vi "DualGateSTS.vi"() -> ()   [LabVIEW 2021]
panel:
  in  "Tabs":enum32{"Main", "Attributes"}(tab)
  in  "Start Gate 1 (V)":dbl
  in  "End Gate 1 (V)":dbl
  in  "Increment Gate 1 (V)":dbl
  in  "Safety Limit 2 (V)":dbl
  in  "Basename":string
  in  "Start Gate 2 (V)":dbl
  in  "End Gate 2 (V)":dbl
  in  "Increment Gate 2 (V)":dbl
  in  "Stop":bool
  out "Current Gate Voltage 2 (V)":dbl
  in  "Attributes":string[][](array[string])
  # "Dual Gate STS"
  # "Gate 2 Parameters"
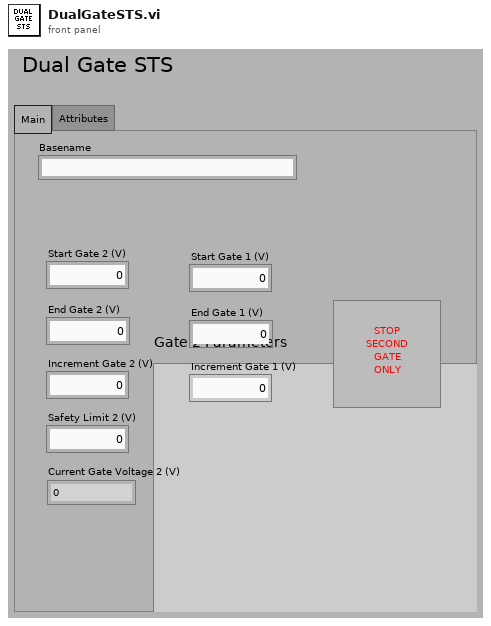
[diagram p1: front panel]
types:
  T1 = enum16{"Output 2 (V)", "Output 3 (V)", "Output 4 (V)"}
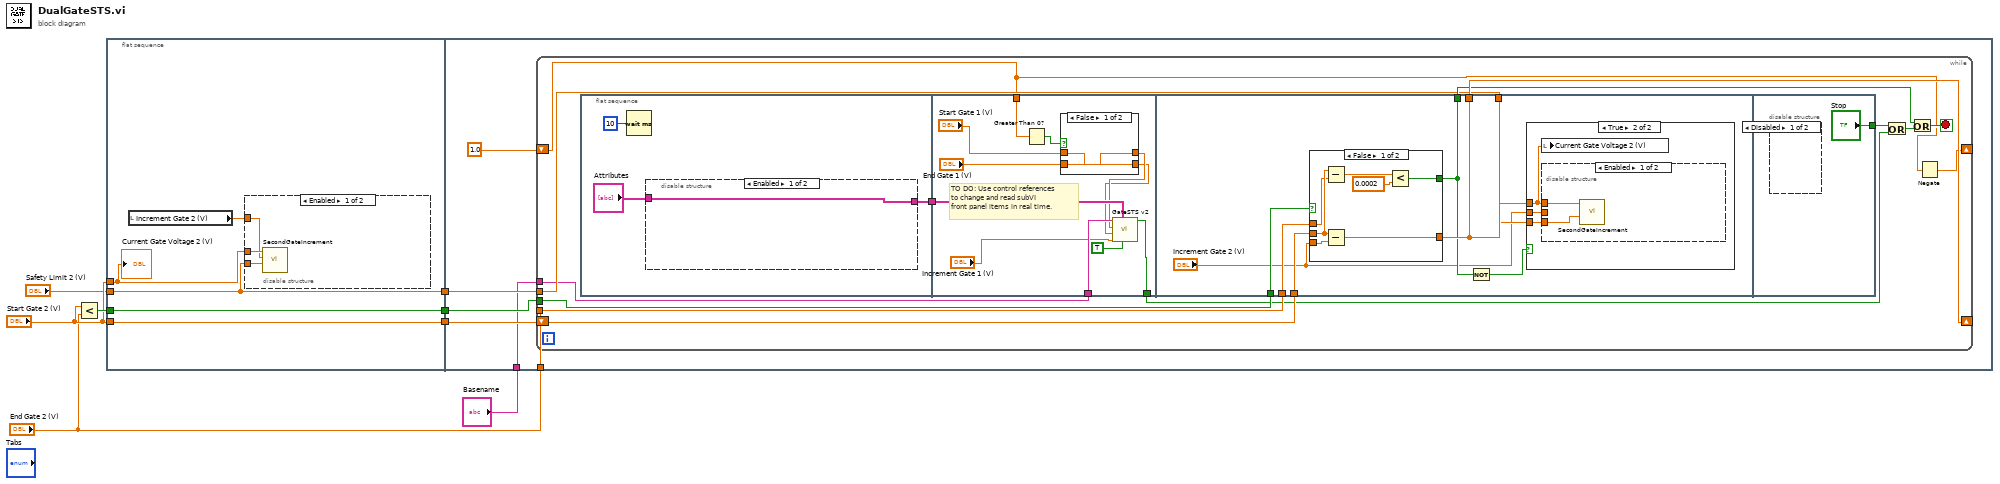
[diagram p0: block diagram]
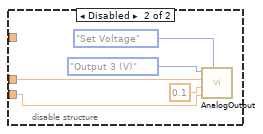
[diagram p2: hidden frame]
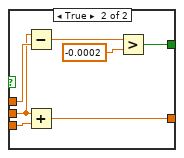
[diagram p5: hidden frame]
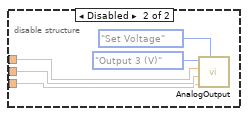
[diagram p7: hidden frame]
diagram:
  n1 = Less?(x="Start Gate 2 (V)", y="End Gate 2 (V)") -> (x < y?=w8:bool)
  n2 = flat-sequence {
    tunnel: [w13] -> w4
    tunnel: [w12] -> w3
    tunnel: [w11] -> w2
    tunnel: "Safety Limit 2 (V)" -> [w11]
    tunnel: "Start Gate 2 (V)" -> [w10]
    tunnel: "Start Gate 2 (V)" -> [w12]
    tunnel: w8 -> [w13]
    tunnel: w4 -> [w27]
    tunnel: w3 -> [w26]
    tunnel: "End Gate 2 (V)" -> [w25]
    tunnel: w2 -> [w24]
    tunnel: "Basename" -> [w23]
    frame #0 {
      n3 = local read "Increment Gate 2 (V)"() -> (w9:dbl)
      n4 = disable-structure shown="Enabled" {
        disable-tunnel: w11 -> [w16 w20]
        disable-tunnel: w10 -> [w15 w21]
        disable-tunnel: w9 -> [w14 _]
        frame Enabled {
          n5 = call "SecondGateIncrement.vi"("Voltage Safety Limit"=w16, "Increment"=w14, "Gate Voltage"=w15) -> ()  [unwired: 9 in]
        }
        frame Disabled {
          n6 = call "AnalogOutput.vi"("Read or Set Voltage?"=enum16{"Read Voltage", "Set Voltage"}."Set Voltage", "Voltage Safety Limit"=w20, "Increment"=0.1, "Target Voltage"=w21, "Channel"=T1."Output 3 (V)") -> ()  [unwired: 6 in, 1 out]
        }
      }
      "Current Gate Voltage 2 (V)" <- w10
    }
    frame #1 {
      n7 = while {
        tunnel: w27 -> [w36]
        shift-right: [w40] -> _
        shift-left: w26 -> [w38]
        tunnel: w25 -> [w37]
        tunnel: w24 -> [w35]
        tunnel: w23 -> [w34]
        shift-right: [w28] -> _
        shift-left: 1.0 -> [w29]
        stop <- w41 stop-if-true
        n8 = flat-sequence {
          tunnel: [w42] -> w33
          tunnel: w34 -> [w56]
          tunnel: w33 -> [w57]
          tunnel: [w54] -> w32
          tunnel: w29 -> [w48]
          tunnel: [w69] -> w40
          tunnel: [w68] -> w39
          tunnel: w38 -> [w67]
          tunnel: w37 -> [w66]
          tunnel: w36 -> [w65]
          tunnel: w35 -> [w63]
          tunnel: ["Stop"] -> w30
          frame #0 {
            n9 = Wait (ms)(milliseconds to wait=u32 10) -> ()  [unwired: 1 out]
            n10 = disable-structure shown="Enabled" {
              disable-tunnel: "Attributes" -> [w45 w46]
              disable-tunnel: [w45 w46] -> w42
              frame Enabled {
              }
              frame Disabled {
              }
            }
          }
          frame #1 {
            # "TO DO: Use control references\nto change and read subVI\nfront panel items in real time."
            n11 = Greater Than 0?(x=w48) -> (x > 0?=w47:bool)
            n12 = case shown="False" w47 {
              tunnel: "Start Gate 1 (V)" -> [w59 w61]
              tunnel: "End Gate 1 (V)" -> [w58 w60]
              tunnel: [w58 w61] -> w50
              tunnel: [w59 w60] -> w49
              frame False {
              }
              frame True {
              }
            }
            n13 = call "GateSTS v2.vi"("Store\nSecond Gate?"=TRUE ("Store\nSecond Gate?"), "Attributes"=w57, "Increment Gate (V)"="Increment Gate 1 (V)", "End Gate (V)"=w49, "Start Gate (V)"=w50, "Basename"=w56) -> ("Stop Loop"=w54:bool)  [unwired: 4 in]
          }
          frame #2 {
            n14 = case shown="False" w65 {
              tunnel: w67 -> [w74 w80]
              tunnel: "Increment Gate 2 (V)" -> [w75 w83]
              tunnel: [w76 w82] -> w69
              tunnel: w66 -> [w73 w81]
              tunnel: [w71 w79] -> w68
              frame False {
                n15 = Subtract(x=w74, y=w73) -> (x-y=w72:dbl)
                n16 = Subtract(x=w74, y=w75) -> (x-y=w76:dbl)
                n17 = Less?(x=w72, y=0.0002) -> (x < y?=w71:bool)
              }
              frame True {
                n18 = Subtract(x=w80, y=w81) -> (x-y=w78:dbl)
                n19 = Add(x=w80, y=w83) -> (x+y=w82:dbl)
                n20 = Greater?(x=w78, y=-0.0002) -> (0:w79:bool)
              }
            }
            n21 = Not(x=w68) -> (.not. x?=w64:bool)
            n22 = case shown="True" w64 {
              tunnel: w69 -> [_ w86]
              tunnel: w63 -> [_ w85]
              tunnel: "Increment Gate 2 (V)" -> [_ w84]
              frame False {
              }
              frame True {
                n23 = local write "Current Gate Voltage 2 (V)"(w86) -> ()
                n24 = disable-structure shown="Enabled" {
                  disable-tunnel: w86 -> [w88 w93]
                  disable-tunnel: w85 -> [w87 w91]
                  disable-tunnel: w84 -> [_ w92]
                  frame Enabled {
                    n25 = call "SecondGateIncrement.vi"("Voltage Safety Limit"=w87, "Gate Voltage"=w88) -> ()  [unwired: 10 in]
                  }
                  frame Disabled {
                    n26 = call "AnalogOutput.vi"("Read or Set Voltage?"=enum16{"Read Voltage", "Set Voltage"}."Set Voltage", "Voltage Safety Limit"=w91, "Increment"=w92, "Target Voltage"=w93, "Channel"=T1."Output 3 (V)") -> ()  [unwired: 6 in, 1 out]
                  }
                }
              }
            }
          }
          frame #3 {
            n27 = disable-structure shown="Disabled" {
              frame Disabled {
              }
              frame Enabled {
              }
            }
          }
        }
        n28 = Or(x=w30, y=w32) -> (x .or. y?=w31:bool)
        n29 = Or(x=w39, y=w31) -> (x .or. y?=w41:bool)
        n30 = Negate(x=w29) -> (-x=w28:dbl)
      }
    }
  }
